vi "Destroy REST Client.vi"(8 "error in (no error)":errorcluster, 11 "REST Client_NET in":refnum<class "REST Client_NET.lvclass">) -> (0 "error out":errorcluster)   [LabVIEW 2018, in "REST Client_NET.lvlib" / "REST Client_NET.lvclass"]
doc: "Destroy REST client reference.\n<b> </b> <b> </b>\nHttpClient_NET\nJustin Young - Viviota\nCopyright (c) 2021\nLicense: BSD"
uses:
  REST Client_NET.lvclass
  REST Client_NET.lvclass/REST Client_NET.ctl
  classes/REST Client/REST Client.lvclass
  LabVIEWHTTPClient_NET/HttpClient_NET.lvclass
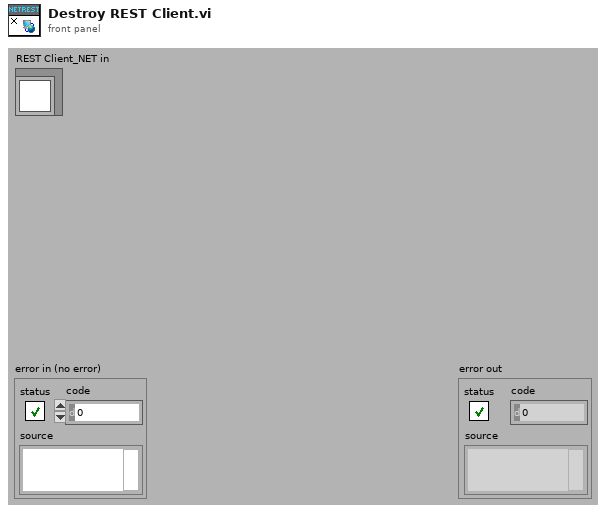
[diagram p1: front panel]
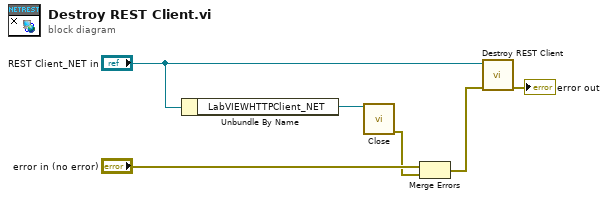
[diagram p0: block diagram]
diagram:
  n1 = Unbundle By Name("REST Client_NET in") -> ("LabVIEWHTTPClient_NET"=w3:refnum<class "HttpClient_NET.lvclass">)
  n2 = call "Close.vi"("LabVIEWHTTPClient_NET in"=w3) -> ("Error Out"=w1:errorcluster)  [unwired: 10 in]
  n3 = Merge Errors("error in (no error)", w1) -> (w2:errorcluster)
  n4 = call-parent "Destroy REST Client.vi"("error in (no error)"=w2, "REST Client in"="REST Client_NET in") -> ("error out"=→"error out":errorcluster)  [unwired: 9 in]
